vi "Sandbox NV.vi"() -> ()   [LabVIEW 2019]
uses:
  NeedleValve_class/NeedleValve.lvclass
  D:/GIT H4000/H4000/src/Device_class/Device.lvclass
  Database_Postgress_class/Database_Postgress.lvclass
  D:/GIT H4000/H4000/src/DatabaseInterface_class/DatabaseInterface.lvclass
  Database_Postgress_class/Connection Info.ctl
  Logger_class/Logger.lvclass
  ConfigJSON_class/ConfigJSON.lvclass
  D:/GIT H4000/H4000/src/ConfigInterface_class/ConfigInterface.lvclass
  FPGA_API_class/FPGA API.lvclass
  Proccess_class/TAGs.ctl
  ConfigJSON_class/ConfigJSON.lvclass/ConfigJSON.ctl
  Proccess_class/Proccess.lvclass/Proccess.ctl
  Device_class/ErrorToDb.vi/d458cff9-8e45-4544-91af-cfa5b3c8a69c.vi
  Proccess_class/GetNames.vi
  Proccess_class/GetLogger.vi
  Device_class/Device.lvclass
  D:/GIT H4000/H4000/src/Proccess_class/Proccess.lvclass
  Logger_class/WriteEvent.vi
  DatabaseInterface_class/DatabaseInterface.lvclass
  SV_Puplisher_class/SV_Publisher.lvclass
  Proccess_class/Proccess.lvclass
panel:
  out "Numeric":i32
  out "Pump_1AI_1DO_2DI out 2":refnum<class "NeedleValve.lvclass">
  out "error out 4":errorcluster
  out "error out 3":errorcluster
  in  "stop":bool
  out "error out":errorcluster
  out "Pump_1AI_1DO_2DI out":refnum<class "NeedleValve.lvclass">
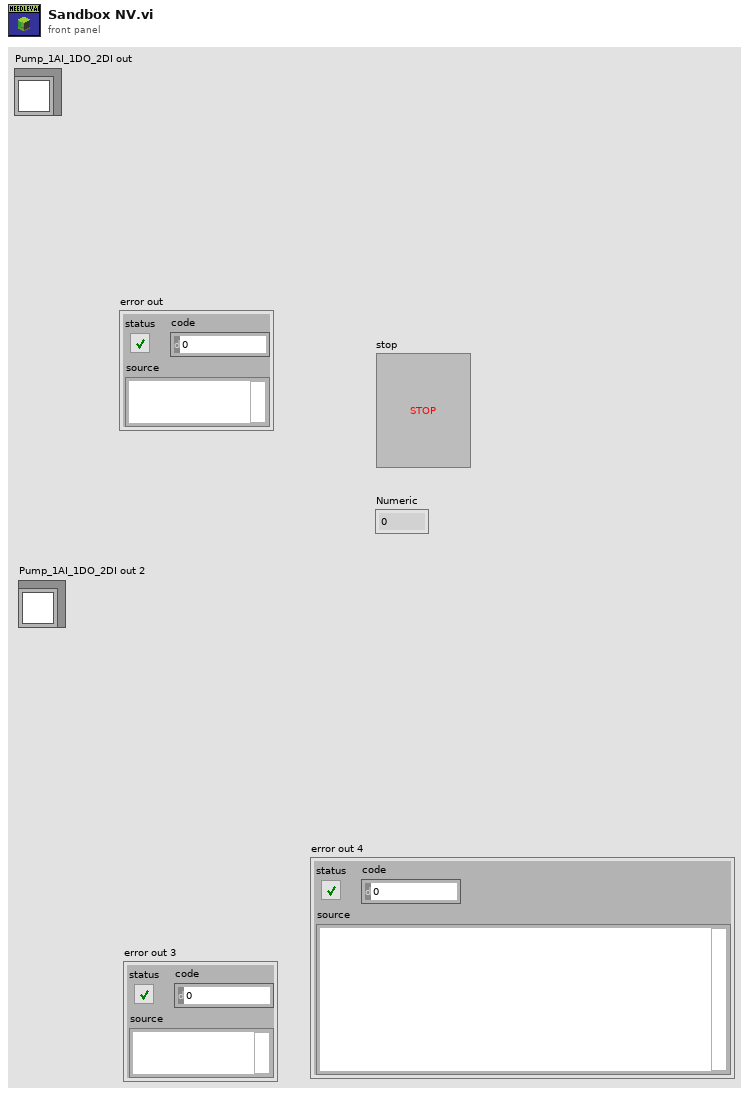
[diagram p1: front panel]
types:
  T1 = typedef "Proccess.lvclass/TAGs.ctl" = cluster{"TAG":string, "PTAG":string, "DESC":string}
  T2 = typedef "DatabaseInterface.lvclass/Connection Info.ctl" = cluster{"IP_Address":string, "Port":u16, "Timeout":i32, "User":string, "Password":string, "Database":string}
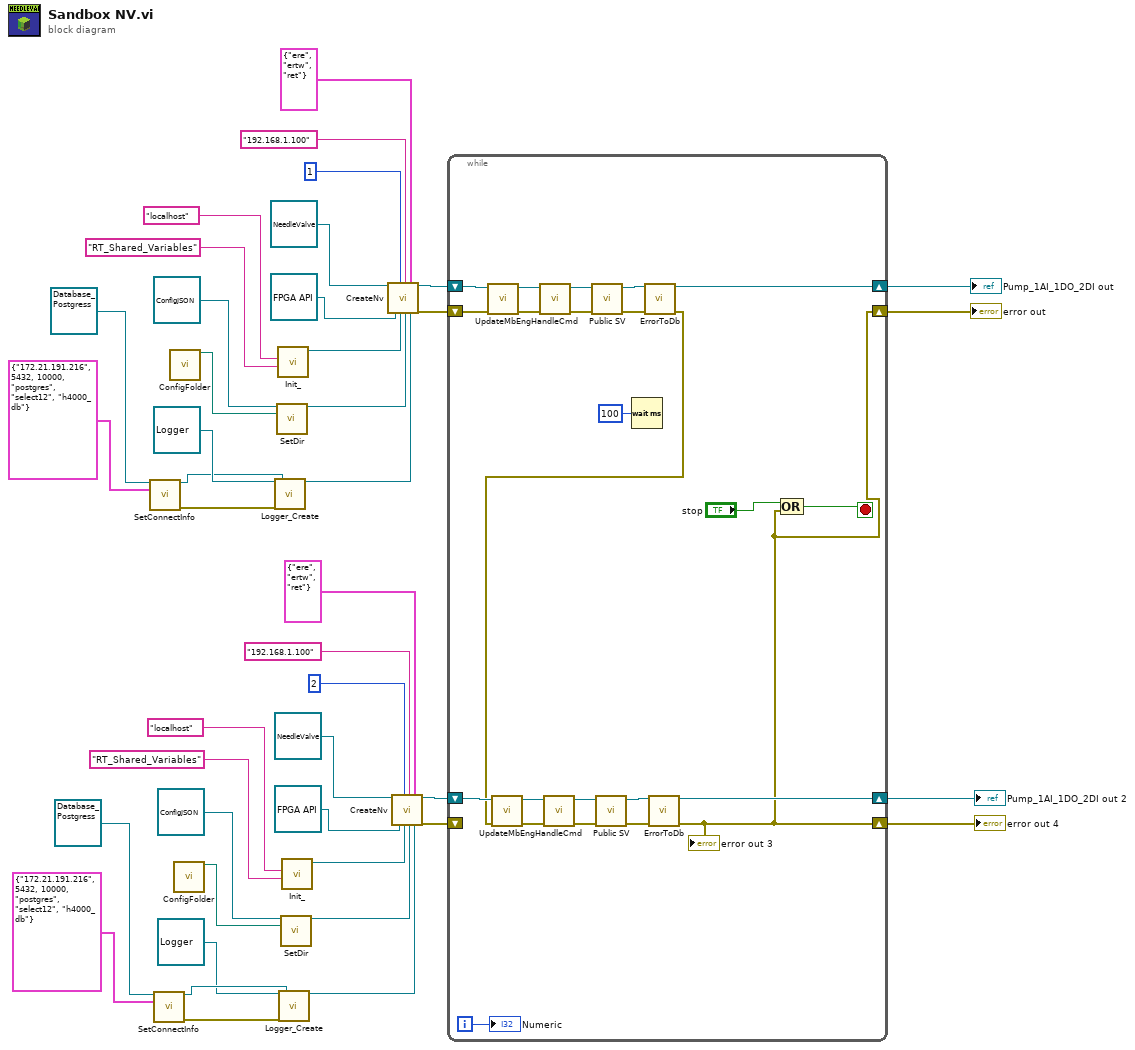
[diagram p0: block diagram]
diagram:
  n1 = call-dynamic "SetConnectInfo.vi"("reference in"=refnum<class "Database_Postgress.lvclass"> refnum, "Connection Info"=T2 {"IP_Address"="172.21.191.216", "Port"=5432, "Timeout"=10000, "User"="postgres", "Password"="select12", "Database"="h4000_db"}) -> ("reference out"=w39:refnum<class "Database_Postgress.lvclass">, "error out"=w38:errorcluster)  [unwired: 12 in]
  n2 = call-dynamic "SetConnectInfo.vi"("reference in"=refnum<class "Database_Postgress.lvclass"> refnum, "Connection Info"=T2 {"IP_Address"="172.21.191.216", "Port"=5432, "Timeout"=10000, "User"="postgres", "Password"="select12", "Database"="h4000_db"}) -> ("reference out"=w4:refnum<class "Database_Postgress.lvclass">, "error out"=w5:errorcluster)  [unwired: 12 in]
  n3 = call "ConfigFolder.vi"() -> ("dup path"=w36:path)  [unwired: 14 in, 1 out]
  n4 = call "ConfigFolder.vi"() -> ("dup path"=w7:path)  [unwired: 14 in, 1 out]
  n5 = call "Logger_Create.vi"("reference in"=refnum<class "Logger.lvclass"> refnum, "error in (no error)"=w38, "DatabaseInterface"=w39) -> ("reference out"=w30:refnum<class "Logger.lvclass">)  [unwired: 15 in, 1 out]
  n6 = call "SetDir.vi"("reference in"=refnum<class "ConfigJSON.lvclass"> refnum ("ConfigJSON"), "Config Dir"=w36) -> ("JSON"=w28:refnum<class "ConfigJSON.lvclass">)  [unwired: 13 in]
  n7 = call "Init_.vi"("lib"="RT_Shared_Variables", "host"="localhost") -> ("SV_Publisher out"=w31:refnum<class "SV_Publisher.lvclass">)  [unwired: 8 in, 1 out]
  n8 = call "Logger_Create.vi"("reference in"=refnum<class "Logger.lvclass"> refnum, "error in (no error)"=w5, "DatabaseInterface"=w4) -> ("reference out"=w13:refnum<class "Logger.lvclass">)  [unwired: 15 in, 1 out]
  n9 = call "SetDir.vi"("reference in"=refnum<class "ConfigJSON.lvclass"> refnum ("ConfigJSON"), "Config Dir"=w7) -> ("JSON"=w15:refnum<class "ConfigJSON.lvclass">)  [unwired: 13 in]
  n10 = call "Init_.vi"("lib"="RT_Shared_Variables", "host"="localhost") -> ("SV_Publisher out"=w12:refnum<class "SV_Publisher.lvclass">)  [unwired: 8 in, 1 out]
  n11 = call "CreateNv.vi"("NeedleValve in"=refnum<class "NeedleValve.lvclass"> refnum, "FPGA API"=refnum<class "FPGA API.lvclass"> refnum, "addres"=u16 1, "SV_Publisher"=w31, "ip"="192.168.1.100", "ConfigInterface"=w28, "Tags"=T1 {"TAG"="ere", "PTAG"="ertw", "DESC"="ret"}, "Logger"=w30) -> ("NeedleValve out"=w24:refnum<class "NeedleValve.lvclass">, "error out"=w23:errorcluster)  [unwired: 10 in]
  n12 = call "CreateNv.vi"("NeedleValve in"=refnum<class "NeedleValve.lvclass"> refnum, "FPGA API"=refnum<class "FPGA API.lvclass"> refnum, "addres"=u16 2, "SV_Publisher"=w12, "ip"="192.168.1.100", "ConfigInterface"=w15, "Tags"=T1 {"TAG"="ere", "PTAG"="ertw", "DESC"="ret"}, "Logger"=w13) -> ("NeedleValve out"=w19:refnum<class "NeedleValve.lvclass">, "error out"=w20:errorcluster)  [unwired: 10 in]
  n13 = while {
    shift-right: [w65] -> w25
    shift-left: w24 -> [w64]
    shift-right: [w43] -> w22
    shift-left: w23 -> [w63]
    shift-right: [w47] -> w18
    shift-left: w19 -> [w48]
    shift-right: [w43] -> w21
    shift-left: w20 -> [_]
    i -> [w45]
    stop <- w46 stop-if-true
    n14 = call "UpdateMbEng.vi"("error in (no error)"=w63, "NeedleValve in"=w64) -> ("error out"=w62:errorcluster, "NeedleValve out"=w61:refnum<class "NeedleValve.lvclass">)  [unwired: 8 in]
    n15 = call "HandleCmd.vi"("error in (no error)"=w62, "NeedleValve in"=w61) -> ("error out"=w59:errorcluster, "NeedleValve out"=w60:refnum<class "NeedleValve.lvclass">)  [unwired: 8 in]
    n16 = call "Public SV.vi"("error in (no error)"=w59, "NeedleValve in"=w60) -> ("error out"=w57:errorcluster, "NeedleValve out"=w58:refnum<class "NeedleValve.lvclass">)  [unwired: 8 in]
    n17 = Wait (ms)(milliseconds to wait=u32 100) -> ()  [unwired: 1 out]
    n18 = call "ErrorToDb.vi"("reference in"=w58, "error in (no error)"=w57) -> ("reference out"=w65:refnum<class "NeedleValve.lvclass">, "error out"=w44:errorcluster)  [unwired: 12 in]
    n19 = call "UpdateMbEng.vi"("error in (no error)"=w44, "NeedleValve in"=w48) -> ("error out"=w49:errorcluster, "NeedleValve out"=w50:refnum<class "NeedleValve.lvclass">)  [unwired: 8 in]
    n20 = call "HandleCmd.vi"("error in (no error)"=w49, "NeedleValve in"=w50) -> ("error out"=w52:errorcluster, "NeedleValve out"=w51:refnum<class "NeedleValve.lvclass">)  [unwired: 8 in]
    n21 = call "Public SV.vi"("error in (no error)"=w52, "NeedleValve in"=w51) -> ("error out"=w54:errorcluster, "NeedleValve out"=w53:refnum<class "NeedleValve.lvclass">)  [unwired: 8 in]
    n22 = call "ErrorToDb.vi"("reference in"=w53, "error in (no error)"=w54) -> ("reference out"=w47:refnum<class "NeedleValve.lvclass">, "error out"=w43:errorcluster)  [unwired: 12 in]
    "error out 3" <- w43
    n23 = Compound Arithmetic op=OR("stop", w43) -> (w46:bool)
    "Numeric" <- w45
  }
  "Pump_1AI_1DO_2DI out" <- w25
  "error out" <- w22
  "Pump_1AI_1DO_2DI out 2" <- w18
  "error out 4" <- w21
